vi "3.3.vi"() -> ()   [LabVIEW 2020]
panel:
  out "display":dbl[](array[numeric])
  out "XY Graph":cluster{dbl[], dbl[]}(graph)
  in  "b":dbl
  in  "a":dbl
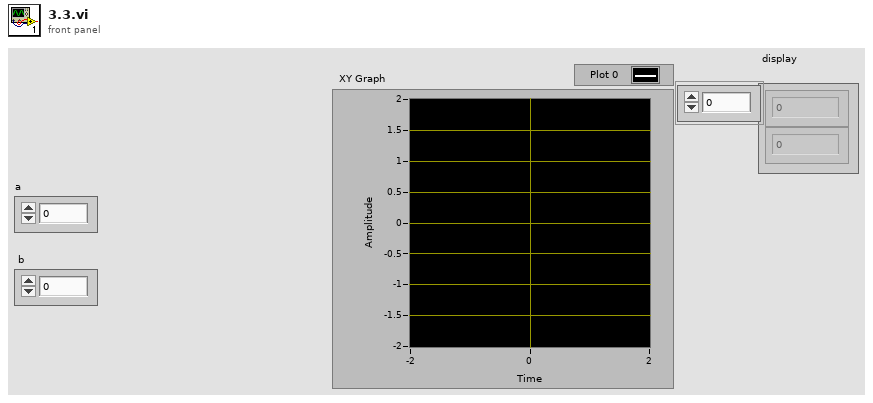
[diagram p1: front panel]
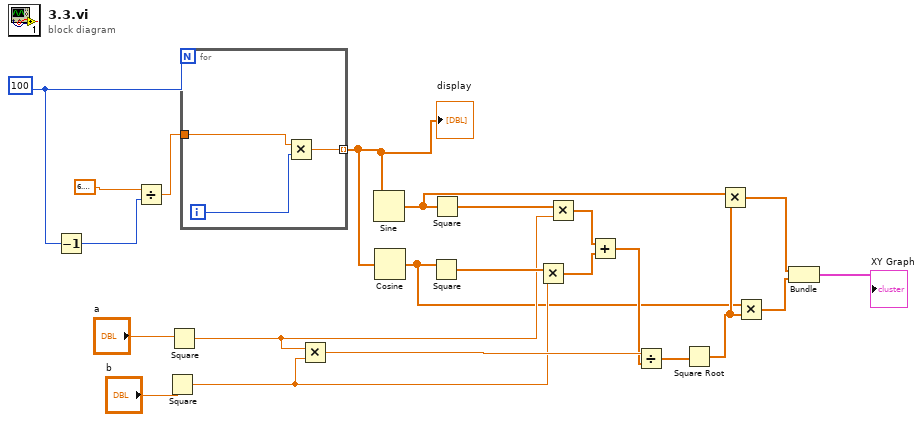
[diagram p0: block diagram]
diagram:
  w4 = 100
  n1 = Decrement(x=w4) -> (x-1=w22:i32)
  n2 = Divide(x=6.283185307179586, y=w22) -> (x/y=w21:dbl)
  n3 = Square(x="b") -> (x^2=w16:dbl)
  n4 = Square(x="a") -> (x^2=w17:dbl)
  n5 = for {
    N: w4 -> [_]
    tunnel: w21 -> [w25]
    tunnel: [w23] -> w6 mode=indexing
    i -> [w24]
    n6 = Multiply(x=w25, y=w24) -> (x*y=w23:dbl)
  }
  "display" <- w6
  n7 = Multiply(x=w17, y=w16) -> (x*y=w18:dbl)
  n8 = Sine(x=w6) -> (sin(x)=w11:dbl[])
  n9 = Cosine(x=w6) -> (cos(x)=w9:dbl[])
  n10 = Square(x=w9) -> (x^2=w19:dbl[])
  n11 = Square(x=w11) -> (x^2=w20:dbl[])
  n12 = Multiply(x=w19, y=w16) -> (x*y=w14:dbl[])
  n13 = Multiply(x=w20, y=w17) -> (x*y=w15:dbl[])
  n14 = Add(x=w15, y=w14) -> (x+y=w13:dbl[])
  n15 = Divide(x=w18, y=w13) -> (x/y=w12:dbl[])
  n16 = Square Root(x=w12) -> (sqrt(x)=w10:dbl[])
  n17 = Multiply(x=w11, y=w10) -> (x*y=w3:dbl[])
  n18 = Multiply(x=w9, y=w10) -> (x*y=w2:dbl[])
  n19 = Bundle(w3, w2) -> (→"XY Graph":cluster{dbl[], dbl[]})  [unwired: 1 in]
